vi "h5_proceed_with_path.vi"(8 "Error in":errorcluster caption="Error in (no error)", 9 "name of caller in":string, 11 "path in":path) -> (0 "Error out":errorcluster, 1 "proceed?":bool, 2 "mode":T1, 3 "path out":path)   [LabVIEW 2015]
uses:
  <vilib>/addons/h5labview2/file/H5Fmode.ctl
  <userlib>/_OpenG.lib/file/file.llb/Valid Path - Traditional__ogtk.vi
  <userlib>/_OpenG.lib/file/file.llb/File Exists - Scalar__ogtk.vi
  <userlib>/_OpenG.lib/file/file.llb/Strip Path Extension - Path__ogtk.vi
  <vilib>/addons/h5labview2/file/H5F.lvlib
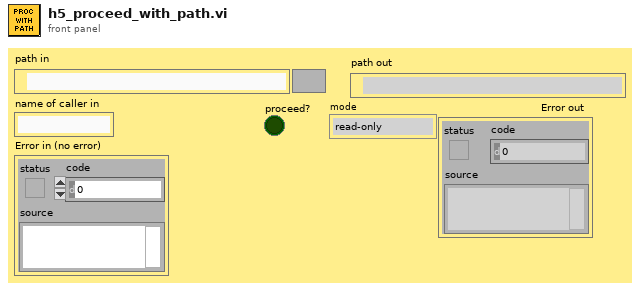
[diagram p1: front panel]
types:
  T1 = typedef "H5F.lvlib/H5Fmode.ctl" = enum16{"read-only", "read-write", "overwrite", "create new", "open or create"}
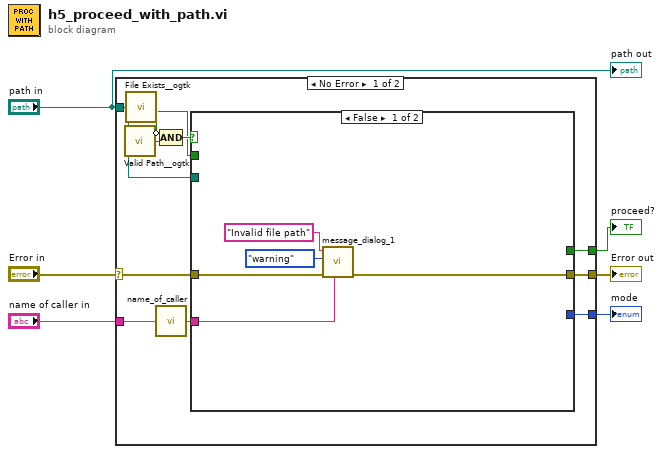
[diagram p0: block diagram]
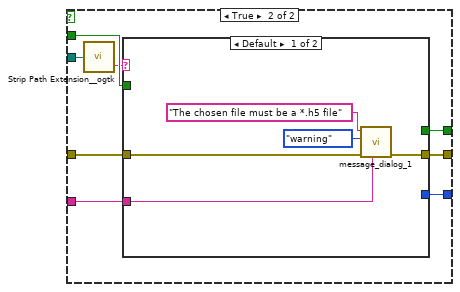
[diagram p2: hidden frame]
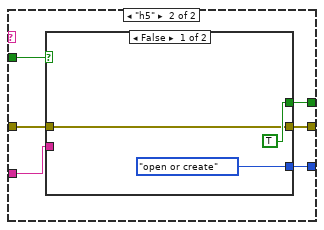
[diagram p3: hidden frame]
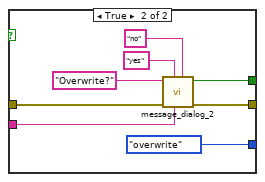
[diagram p4: hidden frame]
diagram:
  n1 = case shown="No Error" "Error in" {
    selector: "Error in" -> [w7 w53]
    tunnel: [w17 _] -> w6
    tunnel: "path in" -> [w12 _]
    tunnel: "name of caller in" -> [w10 _]
    tunnel: [w9 _] -> w3
    tunnel: [w8 w53] -> w2
    frame No Error {
      n2 = call-poly <userlib>:"Valid Path__ogtk.vi"("path"=w12) -> ("valid"=w16:bool)
      n3 = call-poly <userlib>:"File Exists__ogtk.vi"("file path"=w12) -> ("is directory"=w14:bool, "exists"=w13:bool)  [unwired: 6 in]
      n4 = call "name_of_caller.vi"("name of caller in"=w10) -> ("name of caller out"=w11:string)  [unwired: 3 in]
      n5 = Compound Arithmetic op=AND(invert w14, w16) -> (w15:bool)
      n6 = case shown="False" w15 {
        tunnel: [_ w30] -> w17
        tunnel: w13 -> [_ w29]
        tunnel: w12 -> [_ w28]
        tunnel: w11 -> [w20 w26]
        tunnel: [_ w25] -> w9
        tunnel: w7 -> [w19 w24]
        tunnel: [w18 w23] -> w8
        frame False {
          n7 = call "message_dialog_1.vi"("name of caller in"=w20, "Error in"=w19, "flavour (warning)"=enum16{"error", "warning", "message"}."warning" ("flavour (error)"), "text in"="Invalid file path" ("message")) -> ("Error out"=w18:errorcluster)  [unwired: 7 in]
        }
        frame True {
          n8 = call-poly <userlib>:"Strip Path Extension__ogtk.vi"("path"=w28) -> ("extension"=w27:string)  [unwired: 1 out]
          n9 = case shown="Default" w27 {
            tunnel: [_ w41] -> w30
            tunnel: w29 -> [_ w40]
            tunnel: w26 -> [w33 w39]
            tunnel: [_ w38] -> w25
            tunnel: w24 -> [w32 w37]
            tunnel: [w31 w36] -> w23
            frame Default {
              n10 = call "message_dialog_1.vi"("name of caller in"=w33, "Error in"=w32, "flavour (warning)"=enum16{"error", "warning", "message"}."warning" ("flavour (error)"), "text in"="The chosen file must be a *.h5 file") -> ("Error out"=w31:errorcluster)  [unwired: 7 in]
            }
            frame "h5" {
              n11 = case shown="False" w40 {
                tunnel: [TRUE w51] -> w41
                tunnel: w39 -> [_ w48]
                tunnel: [H5Fmode."open or create" ("mode (read-only)") H5Fmode."overwrite" ("mode (read-only)")] -> w38
                tunnel: w37 -> [w42 w46]
                tunnel: [w42 w45] -> w36
                frame False {
                }
                frame True {
                  n12 = call "message_dialog_2.vi"("(CANCEL) button text"="no" ("F button name (\"Cancel\")"), "name of caller in"=w48, "(OK) button text"="yes" ("T button name (\"OK\")"), "Error in"=w46, "text in"="Overwrite?" ("message")) -> ("Error out"=w45:errorcluster, "ok?"=w51:bool)  [unwired: 5 in]
                }
              }
            }
          }
        }
      }
    }
    frame Error {
    }
  }
  "proceed?" <- w6
  "mode" <- w3
  "Error out" <- w2
  "path out" <- "path in"
